vi "Compare Array Ranges.vi"(10 "Target Range":dbl[](array[numeric]), 11 "Check Range":dbl[](array[numeric])) -> (2 "In Range?":bool)   [LabVIEW 2011]
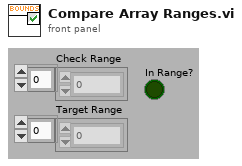
[diagram p1: front panel]
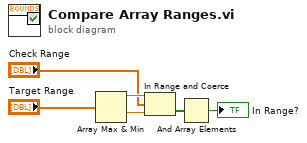
[diagram p0: block diagram]
diagram:
  n1 = Array Max & Min(array="Target Range") -> (max value=w5:dbl, min value=w4:dbl)  [unwired: 2 out]
  n2 = In Range and Coerce(upper limit=w5, x="Check Range", lower limit=w4) -> (In Range?=w2:bool[])  [unwired: 1 out]
  n3 = And Array Elements(Boolean array=w2) -> (logical AND=→"In Range?":bool)
